vi "1D DCT.vi"(10 "DCT size":i32=-1, 11 "X":dbl[](array[numeric])) -> (0 "error":i32, 3 "DCT {X}":dbl[](array[numeric]))   [LabVIEW 2010, in "NI_AALPro.lvlib"]
doc: "Computes the Discrete Cosine Transform (DCT) of the input sequence <B>X</B>. Wire data to the <B>X</B> input to determine the polymorphic instance to use or manually select the instance."
uses:
  NI_AALPro.lvlib
  lvanlys.dll
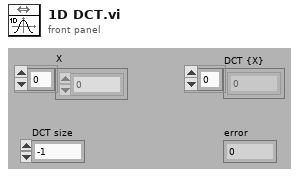
[diagram p1: front panel]
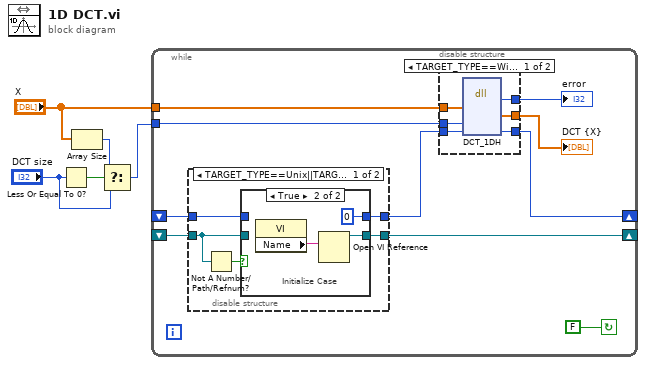
[diagram p0: block diagram]
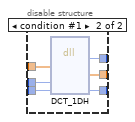
[diagram p2: hidden frame]
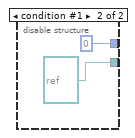
[diagram p4: hidden frame]
diagram:
  n1 = Less Or Equal To 0?(x="DCT size") -> (x <= 0?=w5:bool)
  n2 = Array Size(array="X") -> (size(s)=w2:i32)
  n3 = Select(t=w2, s=w5, f="DCT size") -> (s? t:f=w1:i32)
  n4 = while {
    shift-left: _ -> [w13]
    shift-right: [w7] -> _
    tunnel: "X" -> [w14]
    shift-right: [w12] -> _
    shift-left: _ -> [w11]
    tunnel: w1 -> [w6]
    stop <- FALSE continue-if-true
    n5 = disable-structure shown="TARGET_TYPE==Unix||TARGET_TYPE==Mac||TARGET_TYPE==RT||TARGET_TYPE==Windows, default" {
      disable-tunnel: w11 -> [w30 _]
      disable-tunnel: [w31 refnum<vi> refnum ("VI Refnum")] -> w12
      disable-tunnel: w13 -> [w29 _]
      disable-tunnel: [w28 0 ("t")] -> w8
      frame condition #0 (active) {
        n6 = Not A Number/Path/Refnum?(number/path/refnum=w30) -> (NaN/Path/Refnum?=w32:bool)
        n7 = case shown="True" w32 {
          tunnel: [w34 w37] -> w31
          tunnel: w30 -> [w34 _]
          tunnel: w29 -> [w33 _]
          tunnel: [w33 0 ("error")] -> w28
          frame False {
          }
          frame True {
            # "Initialize Case"
            n8 = property class="VI"() -> ("Name"=w35:string)  [unwired: 2 in, 2 out]
            n9 = Open VI Reference(vi path=w35) -> (vi reference=w37:refnum<vi>)  [unwired: 5 in, 1 out]
          }
        }
      }
      frame condition #1 {
      }
    }
    n10 = disable-structure shown="TARGET_TYPE==Windows||TARGET_TYPE==Mac||TARGET_TYPE==Unix" {
      disable-tunnel: w14 -> [w21 w27]
      disable-tunnel: [w20 w26] -> w10
      disable-tunnel: [w19 w25] -> w9
      disable-tunnel: w8 -> [w18 w24]
      disable-tunnel: [w17 w23] -> w7
      disable-tunnel: w6 -> [w16 w22]
      frame condition #0 (active) {
        n11 = dll-call lib="C:/Program Files/National Instruments/LabVIEW 2010/resource/lvanlys.dll" fn="DCT_1DH"("xH"=w21, "DCTSize"=w16, "tbl"=w18) -> ("return type"=w20:i32, "yH"=w19:dbl[], "tbl"=w17:i64)  [unwired: 6 in, 2 out]
      }
      frame condition #1 {
        n12 = dll-call lib="C:/Program Files/National Instruments/LabVIEW 2010/resource/lvanlys.*" fn="DCT_1DH"("xH"=w27, "DCTSize"=w22, "tbl"=w24) -> (w26:i32, "yH"=w25:dbl[], "tbl"=w23:i32)  [unwired: 6 in, 2 out]
      }
    }
    "error" <- w10
    "DCT {X}" <- w9
  }
